vi "DoCalcDirection.vi"(8 "error in (no error)":errorcluster, 9 "DirectionY":i8, 10 "DirectionX":i8, 11 "AI_Snake in":refnum<class "AI_Snake.lvclass">) -> (0 "error out":errorcluster, 2 "Direction":T1, 3 "AI_Snake out":refnum<class "AI_Snake.lvclass">)   [LabVIEW 2019, in "RT_Game.lvlib" / "AI_Snake.lvclass"]
uses:
  AI_Snake.lvclass
  C:/Users/FreshBob/Dropbox/VIs/myRIO_GameConsole/RT/RT_Game/Snake/Snake.lvclass
  Snake/Direction.ctl
  Snake/Snake.lvclass/Snake.ctl
  AI_Snake.lvclass/AI_Snake.ctl
  Game/Coordinate.ctl
  Snake/Read Position (Tiles).vi
  Snake/Snake.lvclass
  Game/Game.lvclass
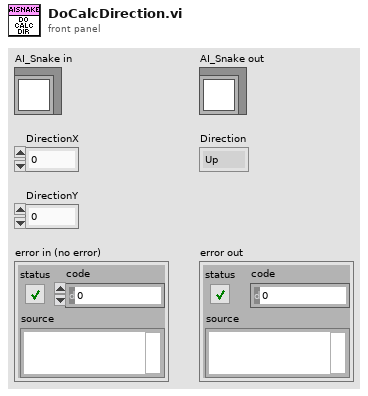
[diagram p1: front panel]
types:
  T1 = typedef "RT_Game.lvlib/Snake.lvclass/Direction.ctl" = enum16{"Up", "Left", "Down", "Right"}
  T2 = typedef "RT_Game.lvlib/Game.lvclass/Coordinate.ctl" = cluster{"x":dbl, "y":dbl}
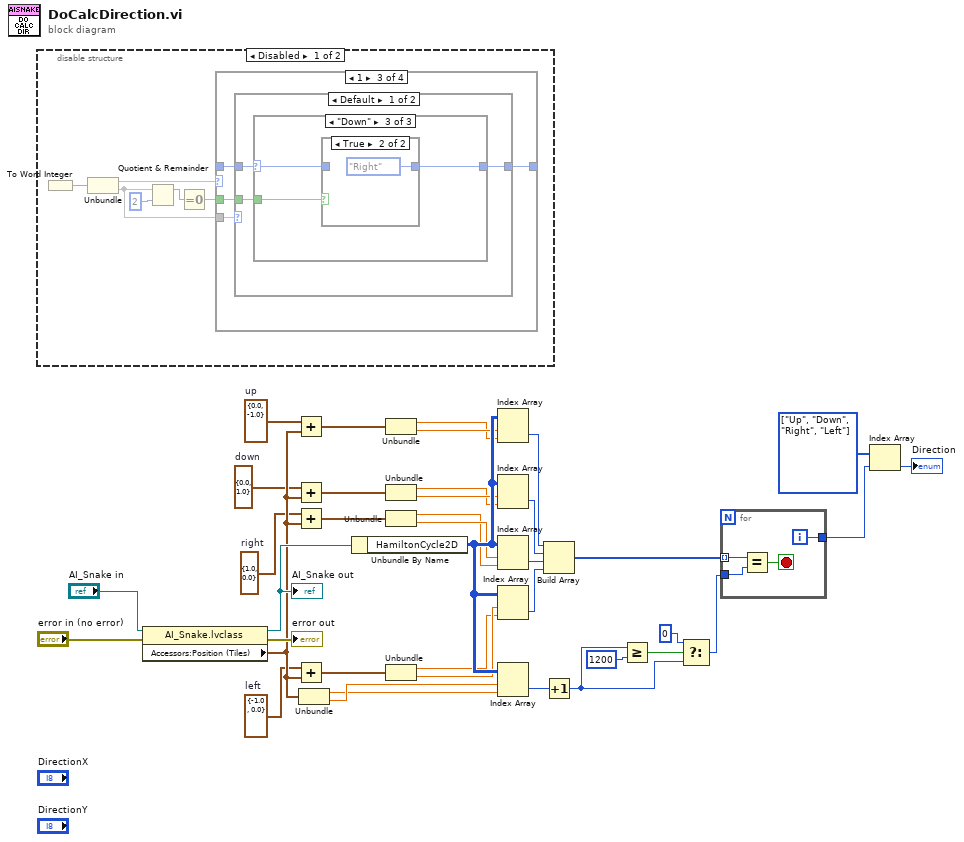
[diagram p0: block diagram]
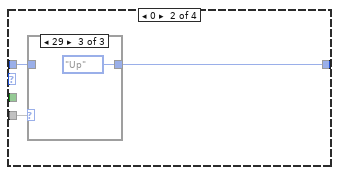
[diagram p3: hidden frame]
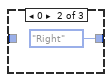
[diagram p5: hidden frame]
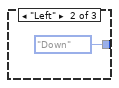
[diagram p7: hidden frame]
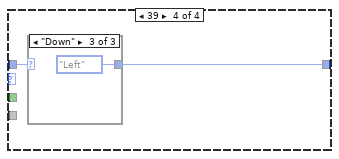
[diagram p10: hidden frame]
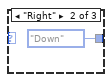
[diagram p12: hidden frame]
diagram:
  w2 = T1[] [enum."Up", enum."Down", enum."Right", enum."Left"] items=["Up", "Left", "Down", "Right"] ("Array")
  w19 = T2 {"x"=0.0, "y"=-1.0}  # up
  w20 = T2 {"x"=0.0, "y"=1.0}  # down
  w21 = T2 {"x"=-1.0, "y"=0.0}  # left
  w22 = T2 {"x"=1.0, "y"=0.0}  # right
  n1 = disable-structure shown="Disabled" {
    frame Disabled {
      n2 = To Word Integer() -> (16bit integer=w39:i16)  [unwired: 1 in]
      n3 = Unbundle(w39) -> (w40, w41)
      n4 = Quotient & Remainder(x=w41, y=i16 2) -> (x-y*floor(x/y)=w43:i16)  [unwired: 1 out]
      n5 = Equal To 0?(x=w43) -> (x = 0?=w44:bool)
      n6 = case shown="1" w40 {
        tunnel: _ -> [w45 w46 w53 w67]
        tunnel: [w45 w47 w54 w68] -> _
        tunnel: w41 -> [_ w48 w55 _]
        tunnel: w44 -> [_ _ w52 _]
        frame Default {
        }
        frame 0 {
          n7 = case shown="29" w48 {
            tunnel: [w49 Direction."Right" ("Direction") Direction."Up" ("Direction")] -> w47
            tunnel: w46 -> [w49 _ _]
            frame Default {
            }
            frame 0 {
            }
            frame 29 {
            }
          }
        }
        frame 1 {
          n8 = case shown="Default" w55 {
            tunnel: [w57 w66] -> w54
            tunnel: w53 -> [w58 w66]
            tunnel: w52 -> [w56 _]
            frame Default {
              n9 = case shown="\"Down\"" w58 {
                selector: w58 -> [w59 _ w62]
                tunnel: [w59 Direction."Down" ("Direction") w63] -> w57
                tunnel: w56 -> [_ _ w61]
                frame Default {
                }
                frame "Left" {
                }
                frame "Down" {
                  n10 = case shown="True" w61 {
                    tunnel: [w64 Direction."Right" ("Direction")] -> w63
                    tunnel: w62 -> [w64 _]
                    frame False {
                    }
                    frame True {
                    }
                  }
                }
              }
            }
            frame 29 {
              # "left"
            }
          }
        }
        frame 39 {
          n11 = case shown="\"Down\"" w67 {
            selector: w67 -> [w69 _ _]
            tunnel: [w69 Direction."Down" ("Direction") Direction."Left" ("Direction")] -> w68
            frame Default {
            }
            frame "Right" {
            }
            frame "Down" {
            }
          }
        }
      }
    }
    frame Enabled {
    }
  }
  n12 = property class="AI_Snake.lvclass"(reference="AI_Snake in", error in="error in (no error)") -> (reference out=w35:refnum<class "AI_Snake.lvclass">, error out=→"error out":errorcluster, "Accessors:Position (Tiles)"=w25:T2)
  "AI_Snake out" <- w35
  n13 = Add(x=w19, y=w25) -> (x+y=w7:T2)
  n14 = Add(x=w20, y=w25) -> (x+y=w6:T2)
  n15 = Add(x=w22, y=w25) -> (x+y=w4:T2)
  n16 = Add(x=w21, y=w25) -> (x+y=w5:T2)
  n17 = Unbundle(w25) -> ("x"=w33:dbl, "y"=w34:dbl)
  n18 = Unbundle By Name(w35) -> ("HamiltonCycle2D"=w32:u16[][])
  n19 = Unbundle(w7) -> ("x"=w23:dbl, "y"=w24:dbl)
  n20 = Unbundle(w6) -> ("x"=w26:dbl, "y"=w27:dbl)
  n21 = Unbundle(w4) -> ("x"=w30:dbl, "y"=w31:dbl)
  n22 = Unbundle(w5) -> ("x"=w28:dbl, "y"=w29:dbl)
  n23 = Index Array(array=w32, index (row)=w24, index (col)=w23) -> (element=w18:u16)
  n24 = Index Array(array=w32, index (row)=w27, index (col)=w26) -> (element=w17:u16)
  n25 = Index Array(array=w32, index (row)=w31, index (col)=w30) -> (element=w16:u16)
  n26 = Index Array(array=w32, index (row)=w29, index (col)=w28) -> (element=w15:u16)
  n27 = Index Array(array=w32, index (row)=w34, index (col)=w33) -> (element=w13:u16)
  n28 = Build Array(w18, w17, w16, w15) -> (w14:u16[])
  n29 = Increment(x=w13) -> (x+1=w12:u16)
  n30 = Greater Or Equal?(x=w12, y=u16 1200) -> (x >= y?=w8:bool)
  n31 = Select(t=u16 0, s=w8, f=w12) -> (s? t:f=w10:u16)
  n32 = for {
    tunnel: w14 -> [w75] mode=indexing
    tunnel: w10 -> [w73]
    tunnel: [w72] -> w3
    i -> [w72]
    stop <- w74 stop-if-true
    n33 = Equal?(x=w75, y=w73) -> (x = y?=w74:bool)
  }
  n34 = Index Array(array=w2, index=w3) -> (element=→"Direction":T1)
